vi "Barycentric method RT.vi"(8 "Next Amp":dbl, 9 "Max Bin":i32, 10 "Max Amp":dbl, 11 "Prev Amp":dbl) -> (3 "Bin":dbl)   [LabVIEW 2014]
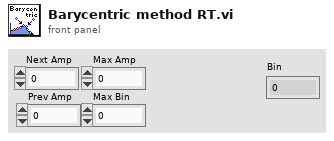
[diagram p1: front panel]
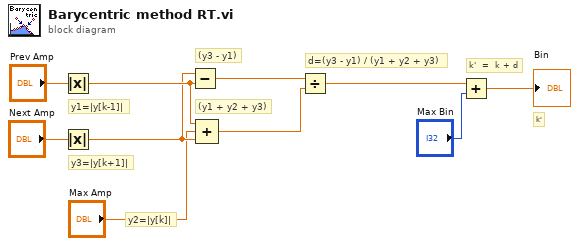
[diagram p0: block diagram]
diagram:
  # "k'"
  # "k'  =  k + d"
  # "d=(y3 - y1) / (y1 + y2 + y3)"
  # "(y1 + y2 + y3)"
  # "(y3 - y1)"
  # "y2=|y[k]|"
  # "y3=|y[k+1]|"
  # "y1=|y[k-1]|"
  n1 = Absolute Value(x="Prev Amp") -> (abs(x)=w10:dbl)
  n2 = Absolute Value(x="Next Amp") -> (abs(x)=w9:dbl)
  n3 = Subtract(x=w9, y=w10) -> (x-y=w8:dbl)
  n4 = Compound Arithmetic op=ADD(w10, "Max Amp", w9) -> (w7:dbl)
  n5 = Divide(x=w8, y=w7) -> (x/y=w6:dbl)
  n6 = Add(x=w6, y="Max Bin") -> (x+y=→"Bin":dbl)
